vi "toml_boolean.vi"(5 "action":T1, 7 "section":string[](array[string]), 8 "error in (no error)":errorcluster, 9 "default":bool, 10 "key":string[](array[string]), 11 "path in":path) -> (0 "error out":errorcluster, 1 "value":bool, 2 "exists?":bool, 3 "path out":path)   [LabVIEW 2017]
uses:
  toml_key_action.ctl
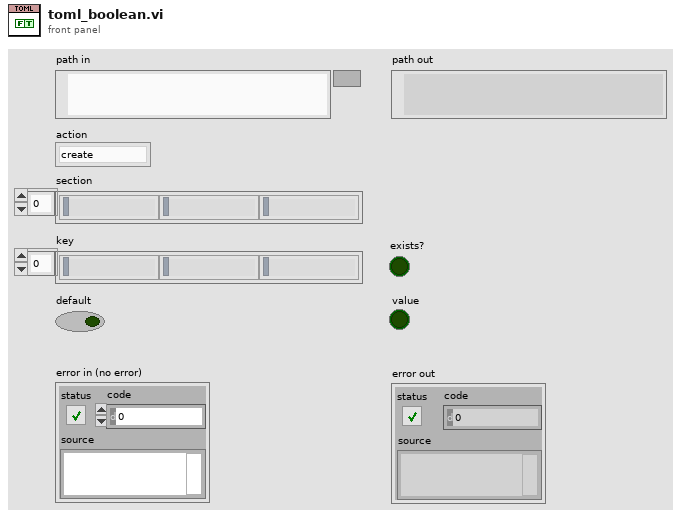
[diagram p1: front panel]
types:
  T1 = typedef "toml_key_action.ctl" = enum8{"create", "read", "write", "delete"}
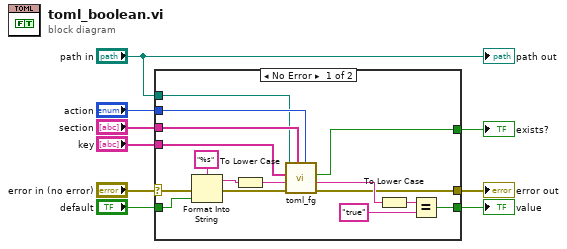
[diagram p0: block diagram]
diagram:
  n1 = case shown="No Error" "error in (no error)" {
    selector: "error in (no error)" -> [w25 w27]
    tunnel: "section" -> [w24 _]
    tunnel: "key" -> [w23 _]
    tunnel: "default" -> [w17 w26]
    tunnel: [w16 w26] -> w5
    tunnel: [w15 w27] -> w4
    tunnel: [w13 _] -> w3
    tunnel: "action" -> [w12 _]
    tunnel: "path in" -> [w11 _]
    frame No Error {
      n2 = Format Into String(format string="%s", error in=w25, w17) -> (resulting string=w20:string, error out=w22:errorcluster)  [unwired: 1 in]
      n3 = To Lower Case(string=w20) -> (all lower case string=w10:string)
      n4 = call "toml_fg.vi"("action"=w12, "section"=w24, "error in (no error)"=w22, "value in"=w10, "key"=w23, "path in"=w11) -> ("error out"=w15:errorcluster, "value out"=w19:string, "exists?"=w13:bool)  [unwired: 1 in, 2 out]
      n5 = To Lower Case(string=w19) -> (all lower case string=w14:string)
      n6 = Equal?(x=w14, y="true") -> (x = y?=w16:bool)
    }
    frame Error {
    }
  }
  "error out" <- w4
  "value" <- w5
  "exists?" <- w3
  "path out" <- "path in"
